vi "Graph Setup.vi"(10 "Graph":refnum<vi>) -> ()   [LabVIEW 2016]
uses:
  <vilib>/Utility/miscctls.llb/LVRectTypeDef.ctl
  <vilib>/picture/picture.llb/Draw True-Color Pixmap.vi
panel:
  out "Value":dbl[][](array[numeric]) format="%.2f"
  out "Total Bounds Rect":T1
  out "Array":dbl[](array[numeric]) format="%.2f"
  in  "Cluster":cluster{"x":i16, "y":i16}
  in  "String":string
  out "Point Horizontals":i32[][](array[numeric])
  out "Y Scale.Range:Increment":dbl
  out "min value":dbl format="%.2f"
  out "max value":dbl format="%.2f"
  out "Y scale max":dbl
  out "Y scale min":dbl
  out "Point Verticals":i32[][](array[numeric])
  out "Text Inserted Vertical":i32[][](array[numeric])
  out "Text Insterted Horizontal":dbl[][](array[numeric])
  out "Plot Area Bounds":T1
  in  "error in (no error)":errorcluster
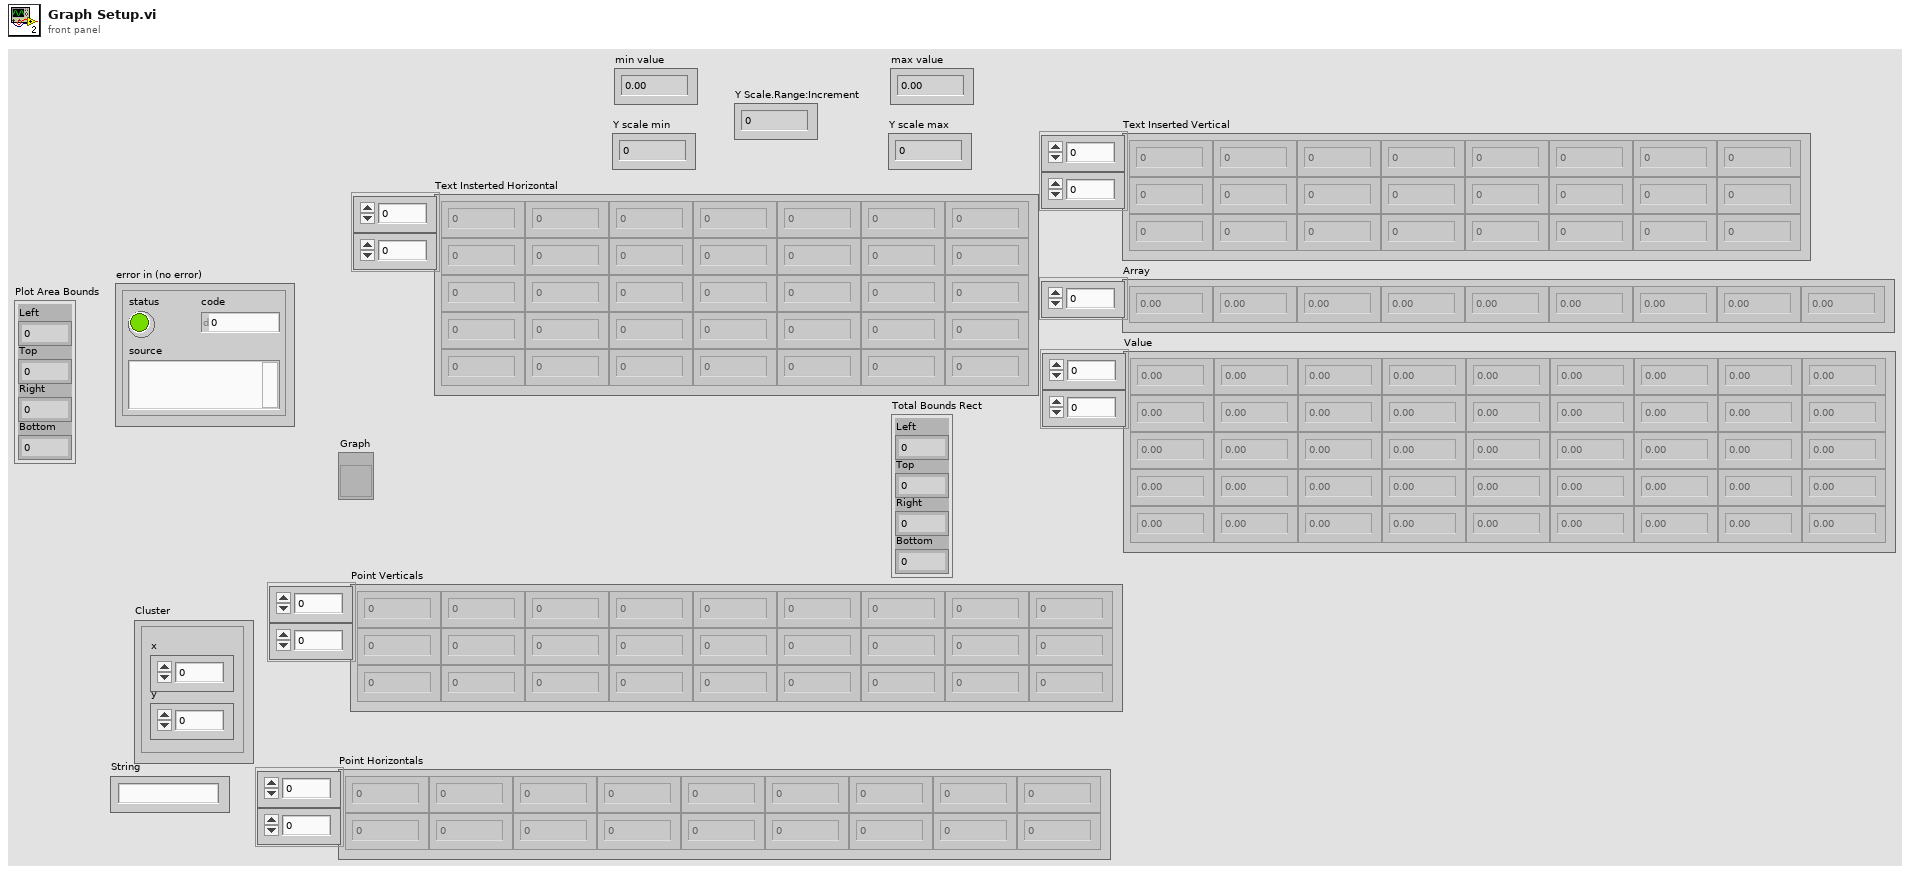
[diagram p1: front panel]
types:
  T1 = typedef "LVRectTypeDef.ctl" = cluster{"Left":i16, "Top":i16, "Right":i16, "Bottom":i16}
  T2 = typedef "LVPoint32TypeDef.ctl" = cluster{"Horizontal":i32, "Vertical":i32}
  T3 = cluster{"left":i16, "top":i16, "right":i16, "bottom":i16}
  T4 = typedef "imagedata.ctl" = cluster{"image type":i32, "image depth":i32, "image":u8[], "mask":u8[], "colors":u32[], "Rectangle":cluster{"left":i16, "top":i16, "right":i16, "bottom":i16}}
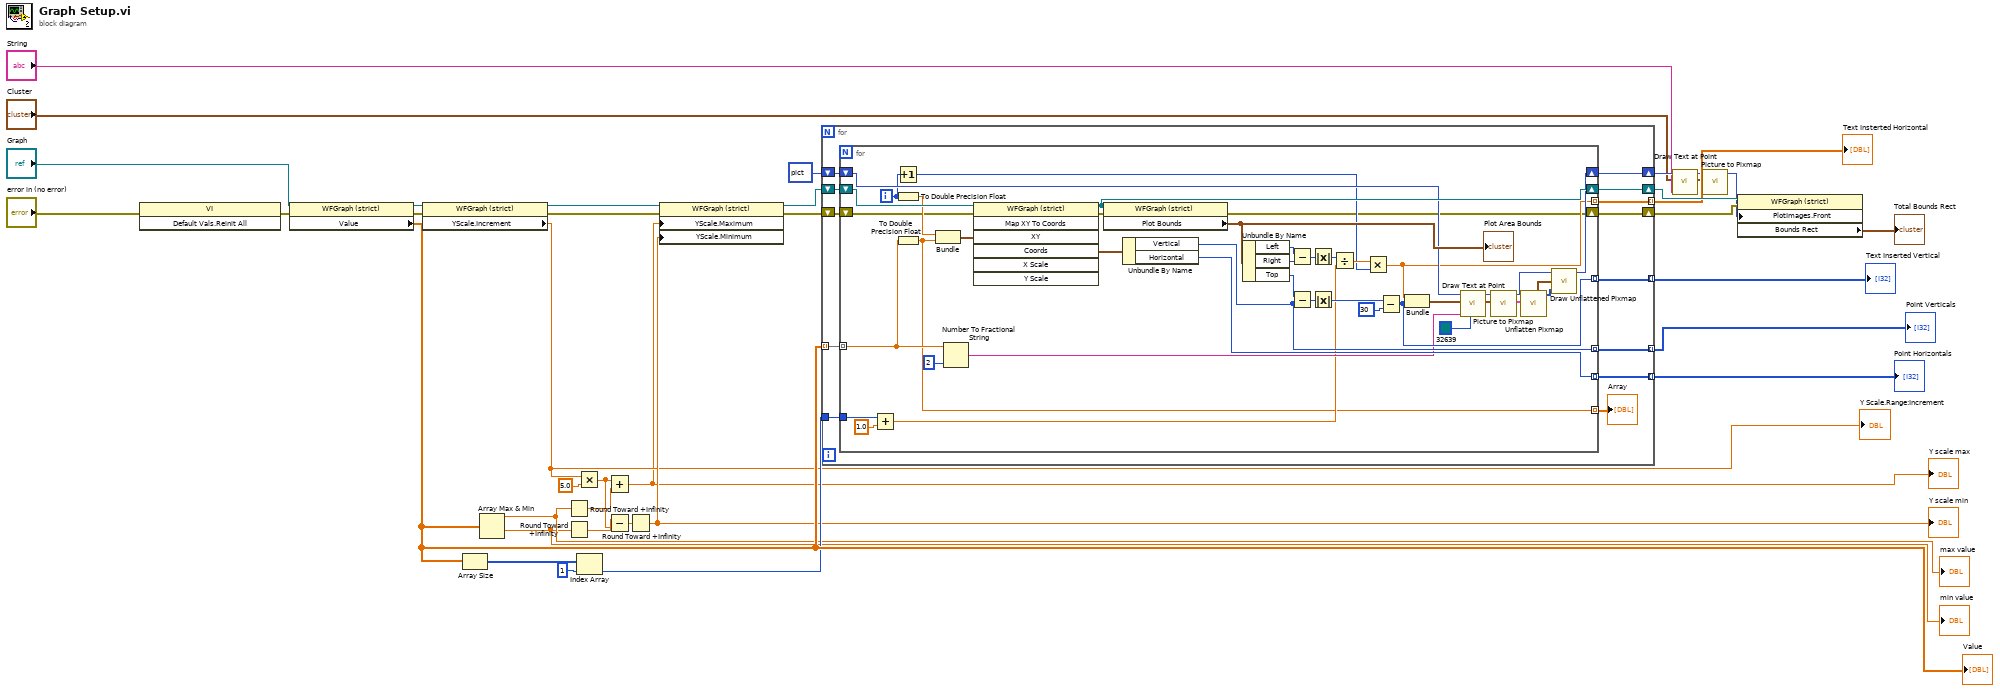
[diagram p0: block diagram]
diagram:
  n1 = invoke class="VI" method="Default Vals.Reinit All"(error in="error in (no error)") -> (error out=w2:errorcluster)  [unwired: 2 in, 2 out]
  n2 = property class="WFGraph (strict)"(reference="Graph", error in=w2) -> (reference out=w35:refnum<vi>, error out=w31:errorcluster, "Value"=w33:dbl[][])
  "Value" <- w33
  n3 = property class="WFGraph (strict)"(reference=w35, error in=w31) -> (reference out=w34:refnum<vi>, error out=w30:errorcluster, "YScale.Increment"=w19:dbl)
  "Y Scale.Range:Increment" <- w19
  n4 = Array Size(array=w33) -> (size(s)=w24:i32[])
  n5 = Array Max & Min(array=w33) -> (max value=w17:dbl, min value=w15:dbl)  [unwired: 2 out]
  "max value" <- w17
  "min value" <- w15
  n6 = Round Toward +Infinity(x=w17) -> (ceil(x): smallest int >= x=w16:dbl)
  n7 = Round Toward +Infinity(x=w15) -> (ceil(x): smallest int >= x=w14:dbl)
  n8 = Multiply(x=w19, y=5.0) -> (x*y=w13:dbl)
  n9 = Index Array(array=w24, index=1) -> (element=w22:i32)
  n10 = Add(x=w13, y=w16) -> (x+y=w12:dbl)
  "Y scale max" <- w12
  n11 = Subtract(x=w14, y=w13) -> (x-y=w21:dbl)
  n12 = Round Toward +Infinity(x=w21) -> (ceil(x): smallest int >= x=w20:dbl)
  "Y scale min" <- w20
  n13 = property class="WFGraph (strict)"(reference=w34, error in=w30, "YScale.Maximum"=w12, "YScale.Minimum"=w20) -> (reference out=w32:refnum<vi>, error out=w29:errorcluster)
  n14 = for {
    tunnel: [w47] -> w26 mode=indexing
    tunnel: [w46] -> w27 mode=indexing
    tunnel: [w45] -> w11 mode=indexing
    tunnel: [w44] -> w25 mode=indexing
    tunnel: w33 -> [w43] mode=indexing
    shift-right: [w48] -> w8
    shift-left: picture data[5B] ("picture") -> [w49]
    shift-right: [w50] -> w37
    shift-left: w32 -> [w42]
    shift-right: [w40] -> w28
    shift-left: w29 -> [w41]
    tunnel: w22 -> [w39]
    n15 = for {
      tunnel: w43 -> [w61] mode=indexing
      shift-right: [w84] -> w50
      shift-left: w42 -> [w91]
      shift-right: [w78] -> w48
      shift-left: w49 -> [w79]
      tunnel: [w69] -> w47 mode=indexing
      tunnel: [w68] -> w46 mode=indexing
      tunnel: [w66] -> w44 mode=indexing
      tunnel: [w65] -> w45 mode=indexing
      tunnel: w39 -> [w58]
      shift-right: [w52] -> w40
      shift-left: w41 -> [w54]
      tunnel: [w51] -> w38 mode=indexing
      i -> [w71]
      n16 = Add(x=w58, y=1.0) -> (x+y=w56:dbl)
      n17 = Increment(x=w71) -> (x+1=w59:i32)
      n18 = To Double Precision Float(number=w71) -> (double precision float=w82:dbl)
      n19 = To Double Precision Float(number=w61) -> (double precision float=w51:dbl)
      n20 = Bundle(w82, w51) -> (w80:cluster{dbl, dbl})  [unwired: 1 in]
      n21 = Number To Fractional String(number=w61, precision (6)=i16 2) -> (F-format string=w62:string)  [unwired: 2 in]
      n22 = invoke class="WFGraph (strict)" method="Map XY To Coords"(reference=w91, error in=w54, "XY"=w80) -> (reference out=w84:refnum<vi>, error out=w53:errorcluster, "Coords"=w81:T2)  [unwired: 4 in, 4 out]
      n23 = property on="Property Node" class="WFGraph (strict)"(reference=w84, error in=w53) -> (error out=w52:errorcluster, "Plot Bounds"=w83:T1)  [unwired: 1 out]
      "Plot Area Bounds" <- w83
      n24 = Unbundle By Name(w81) -> ("Vertical"=w66:i32, "Horizontal"=w65:i32)
      n25 = Unbundle By Name(w83) -> ("Left"=w74:i16, "Right"=w73:i16, "Top"=w77:i16)
      n26 = Subtract(x=w74, y=w73) -> (x-y=w72:i16)
      n27 = Subtract(x=w77, y=w66) -> (x-y=w76:i32)
      n28 = Absolute Value(x=w72) -> (abs(x)=w64:i16)
      n29 = Absolute Value(x=w76) -> (abs(x)=w75:i32)
      n30 = Divide(x=w64, y=w56) -> (x/y=w63:dbl)
      n31 = Multiply(x=w63, y=w59) -> (x*y=w68:dbl)
      n32 = Subtract(x=w75, y=30) -> (x-y=w69:i32)
      n33 = Bundle(w68, w69) -> (w70:cluster{dbl, i32})  [unwired: 1 in]
      n34 = call <vilib>:"Draw Text at Point.vi"("text color(black)"=u32 32639, "text"=w62, "origin"=w70, "picture"=w79) -> ("text rect"=w85:T3, "new picture"=w87:picture)  [unwired: 6 in]
      n35 = call <vilib>:"Picture to Pixmap.vi"("rect"=w85, "picture"=w87) -> ("image data"=w88:T4, "new picture"=w60:picture)  [unwired: 8 in]
      n36 = call <vilib>:"Unflatten Pixmap.vi"("image data"=w88) -> ("24-bit pixmap"=w86:u32[][], "top left"=w90:cluster{"x":i16, "y":i16})  [unwired: 4 in, 5 out]
      n37 = call-poly <vilib>:"Draw Unflattened Pixmap.vi"("picture"=w60, "top left point(0, 0)"=w90, "data (RGB format)"=w86) -> ("new picture"=w78:picture)  [unwired: 6 in]
    }
    "Array" <- w38
  }
  "Text Insterted Horizontal" <- w27
  "Text Inserted Vertical" <- w26
  "Point Verticals" <- w25
  "Point Horizontals" <- w11
  n38 = call <vilib>:"Draw Text at Point.vi"("text"="String", "origin"="Cluster", "picture"=w8) -> ("text rect"=w10:T3, "new picture"=w9:picture)  [unwired: 7 in]
  n39 = call <vilib>:"Picture to Pixmap.vi"("rect"=w10, "picture"=w9) -> ("new picture"=w7:picture)  [unwired: 8 in, 1 out]
  n40 = property on="Property Node" class="WFGraph (strict)"(reference=w37, error in=w28, "PlotImages.Front"=w7) -> ("Bounds Rect"=→"Total Bounds Rect":T1)  [unwired: 2 out]
